vi "rqcBob Channel Test (Low Level Example).vi"() -> ()   [LabVIEW 2019]
uses:
  FPGA/rqcBob/Custom Controls/Pulse Train/rqcBob Pulse Train Config.ctl
  FPGA/rqcBob/Custom Controls/Pulse Train/rqcBob Pulse Train.Generation Mode.ctl
  FPGA/rqcBob/Custom Controls/Pulse Train/rqcBob Pulse Train.First Pulse Delay Mode.ctl
  FPGA/rqcBob/Custom Controls/rqcBob Modulator Config.ctl
  FPGA/rqcBob/Custom Controls/rqcBob Window Config.ctl
  Shared/Shared FPGA Lib/Shared Logic/Custom Controls/rqc Random Generator.parameters.ctl
  Shared/Shared FPGA Lib/Shared Logic/Custom Controls/rqc Random Generator.value type.ctl
  FPGA/rqcBob/Custom Controls/rqcBob Trigger Type.ctl
  <vilib>/FPGAPlugInAG/PCIe-7820R/niLvFpga_Open_PCIe-7820R.vi
  <vilib>/rvi/interface/common/dynamic/niFpgaDynamicAddResources.vi
  Low Level API/Configuration/Photon Detector/Detection FIFOs config/rqcBob Configure PD Detect FIFO (1PD PD1).vi
  Low Level API/Read/Read PD Detection FIFO/rqcBob Read PD Detection FIFO (1PD PD1).vi
  <vilib>/FPGAPlugInAG/Dynamic/niLvFpga_Close_Dynamic.vi
  <vilib>/rvi/interface/nirviOpenFPGA/nirviOpenFPGA.xnode
  FPGA Bitfiles/rqcBob (FPGA) 7820  (MB_SPARTAN7) v 4.0.0.lvbitx.lvbitx
  <vilib>/rvi/interface/nirviCloseFPGA/nirviCloseFPGA.xnode
  <vilib>/Analysis/NI_AALPro.lvlib
panel:
  out "Histogram graph":T1(graph)
  out "Done":bool=TRUE
  in  "stop":bool
  in  "Tab Control":T2(tab)
  in  "train.configuration":T3={"period"=0, "num of pulses"=0, "mode"=enum."train sequence.single", "num of trains"=0, "first pulse delay mode"=enum."every train", "first pulse delay"=55} caption="Pulsed laser configuration"
  in  "modulator.config":T6 caption="Phase modulation"
  in  "window.config":T7 caption="Registration of detector clicks"
  in  "rndGen.parameters":T8={"value type"=enum."constant", "constant"=0, "num of levels"=4, "levels values"=[0, 0, 0, 0]} caption="Phase modulation value" {"num of levels" min=4 max=4 step=1}
  out "Parameters Check Msg":string="Selected parameter combination\nmay lead to inappropriate measurement results"
  in  "Blank Button":bool
  out "sum":i32 caption="Total detector clicks"
  out "DRC":dbl=nan caption="Detection Clicks Rate (Clicks/sec)"
  in  "modulator.clock delay":fxp<+,4,4> caption="PM Clock Delay (0-7) (in units of 40ns)"
  out "SPD.max meas length":u32 caption="SPD max measurement length (in units of 5ns)"
  in  "train.software trigger":bool
  # "Constant"
  # "Random"
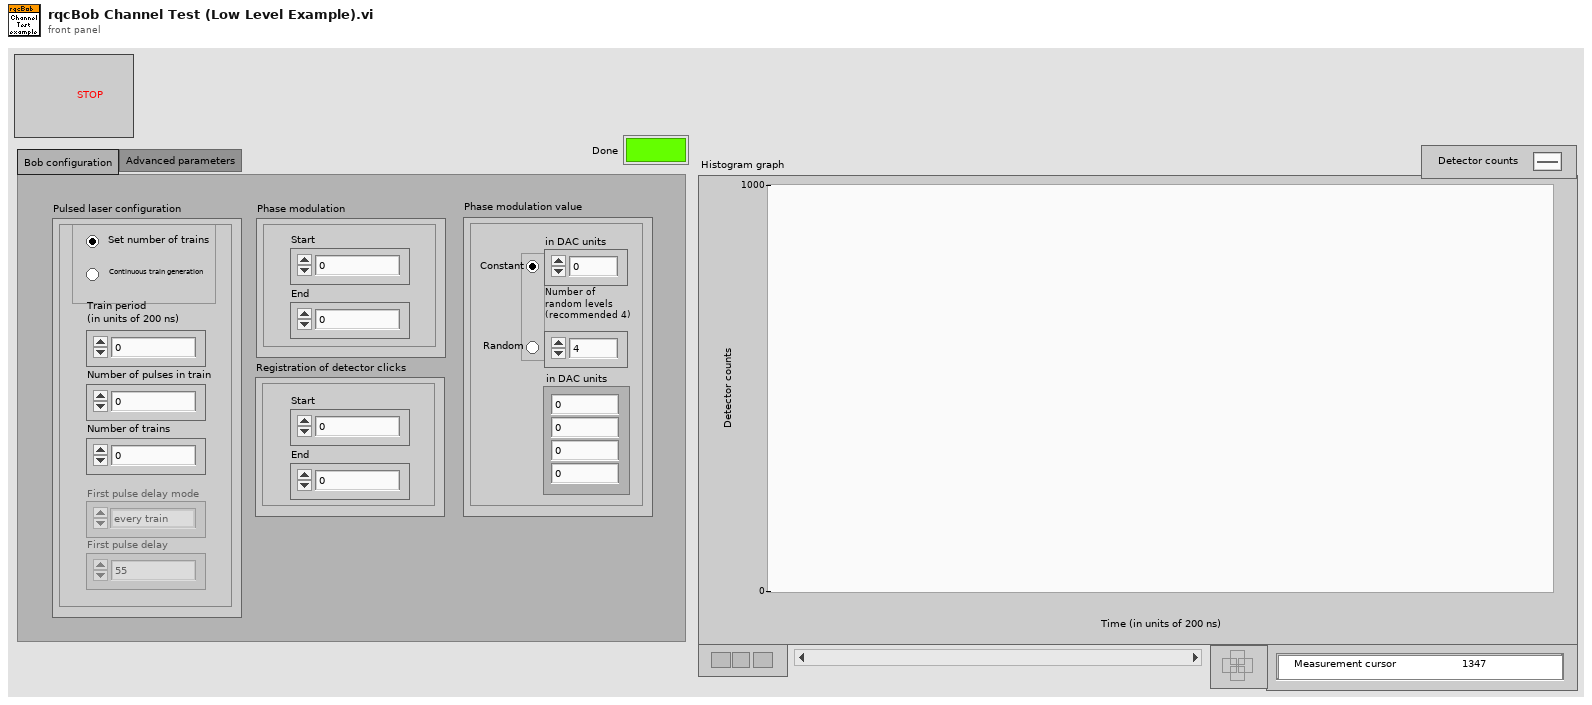
[diagram p1: front panel]
types:
  T1 = cluster{"X Values":dbl[], "Histogram: h(x)":i32[]}
  T2 = enum32{"Bob configuration", "Advanced parameters"}
  T3 = typedef "rqcBob Pulse Train Config.ctl" = cluster{"period":u16, "num of pulses":u16, "mode":T4, "num of trains":u16, "first pulse delay mode":T5, "first pulse delay":u16}
  T4 = typedef "rqcBob Pulse Train.Generation Mode.ctl" = enum32{"single train", "train sequence.single", "train sequence.wait for trigger", "continuous"}
  T5 = typedef "rqcBob Pulse Train.First Pulse Delay Mode.ctl" = enum8{"none", "every train", "first train"}
  T6 = typedef "rqcBob Modulator Config.ctl" = cluster{"modulator.start":u16, "modulator.stop":u16}
  T7 = typedef "rqcBob Window Config.ctl" = cluster{"window.open":u16, "window.close":u16}
  T8 = typedef "rqc Random Generator.parameters.ctl" = cluster{"value type":T9, "constant":u16, "num of levels":u16, "levels values":u16[]}
  T9 = typedef "rqc Random Generator.value type.ctl" = enum32{"random value", "constant"}
  T10 = typedef "rqcBob Trigger Type.ctl" = enum16{"software", "immediate", "DIO"}
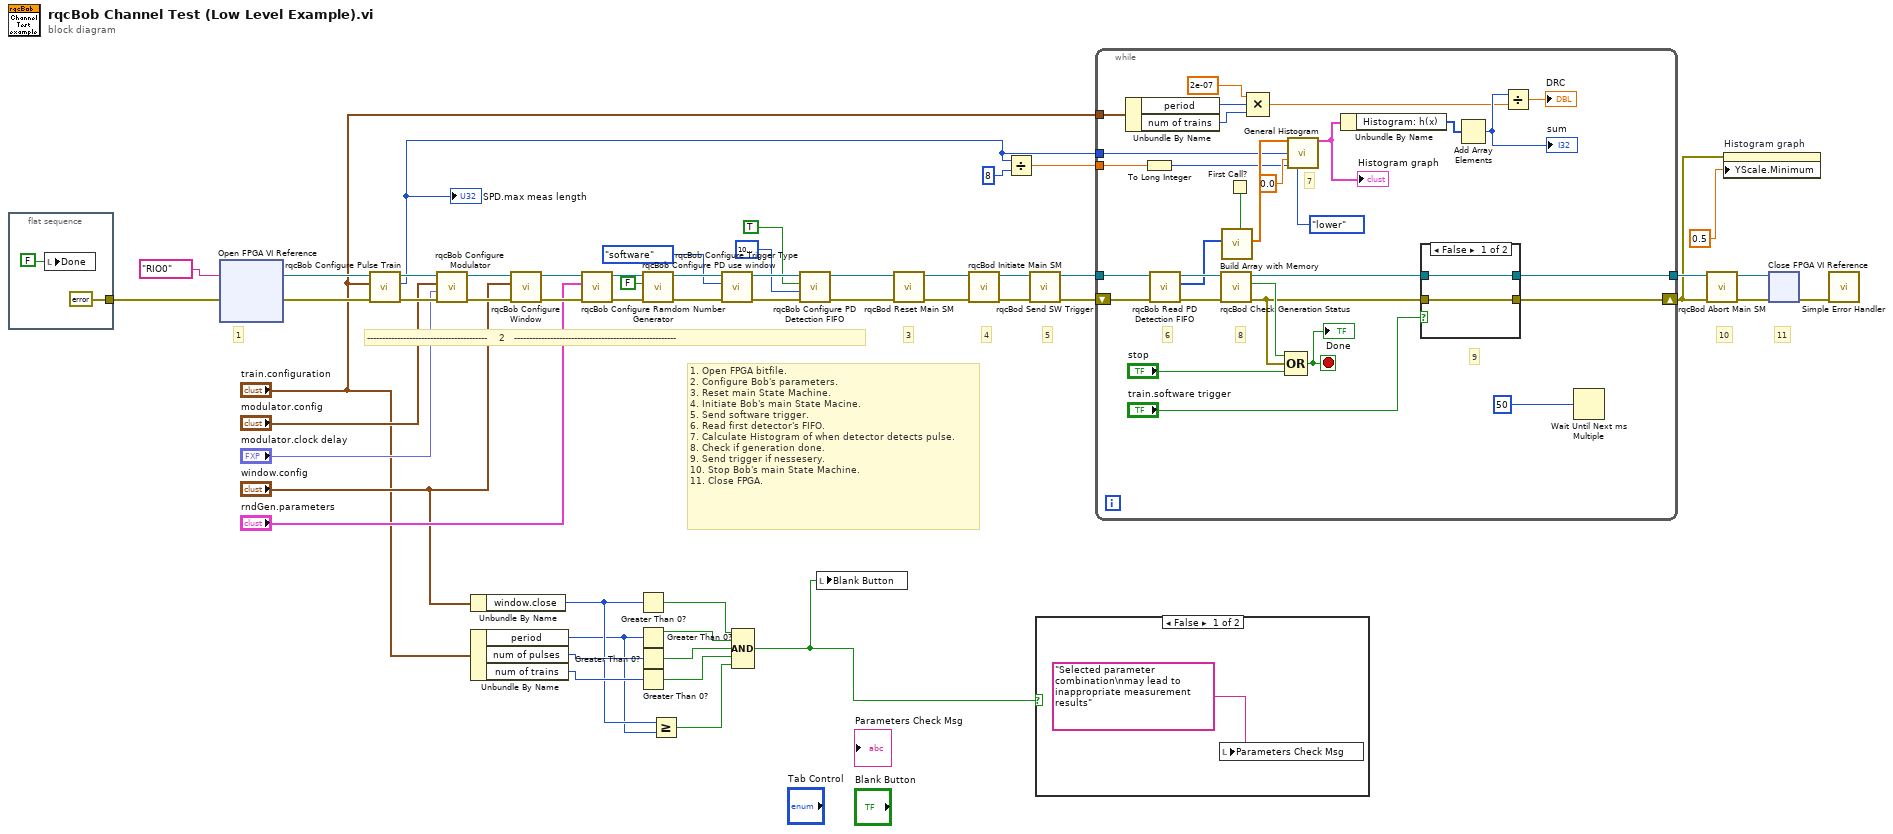
[diagram p0: block diagram]
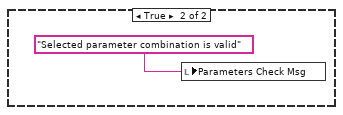
[diagram p2: hidden frame]
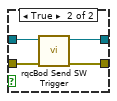
[diagram p3: hidden frame]
diagram:
  # "1. Open FPGA bitfile.\n2. Configure Bob's parameters.\n3. Reset main State Machine.\n4. Initiate Bob's main State Macine.\n5. Send software trigger.\n6. Read first detector's FIFO.\n7. Calculate Histogram of when detector detects pulse.\n8. Check if generation done.\n9. Send trigger if nessesery.\n10. Stop Bob's main State Machine.\n11. Close FPGA."
  # "1"
  # "11"
  # "10"
  # "5"
  # "4"
  # "3"
  # "----------------------------------------    2   ------------------------------------------------------"
  n1 = flat-sequence {
    tunnel: [errorcluster {"status"=FALSE, "code"=0, "source"=""} ("error in")] -> w31
    frame #0 {
      n2 = local write "Done"(FALSE ("Done")) -> ()
    }
  }
  n3 = xnode "Open FPGA VI Reference"("error in"=w31, "resource name"=tag "RIO0") -> ("FPGA VI Reference Out"=w28:refnum<k20>, "error out"=w27:errorcluster)
  n4 = call "rqcBob Configure Pulse Train.vi"("error in"=w27, "train.configuration"="train.configuration", "FPGA reference in"=w28) -> ("error out"=w50:errorcluster, "SPD meas length"=w3:u32, "FPGA reference out"=w51:refnum<k20>)  [unwired: 6 in]
  "SPD.max meas length" <- w3
  n5 = call "rqcBob Configure Modulator.vi"("error in"=w50, "modulator.clock delay"="modulator.clock delay", "modulator.config"="modulator.config", "FPGA reference in"=w51) -> ("error out"=w47:errorcluster, "FPGA reference out"=w48:refnum<k20>)  [unwired: 6 in]
  n6 = Unbundle By Name("window.config") -> ("window.close"=w9:u16)
  n7 = Unbundle By Name("train.configuration") -> ("period"=w8:u16, "num of pulses"=w15:u16, "num of trains"=w14:u16)
  n8 = call "rqcBob Configure Window.vi"("error in"=w47, "window.config"="window.config", "FPGA reference in"=w48) -> ("error out"=w45:errorcluster, "FPGA reference out"=w46:refnum<k20>)  [unwired: 7 in]
  n9 = call "rqcBob Configure Ramdom Number Generator.vi"("error in"=w45, "rqcBob rndGen.parameters"="rndGen.parameters", "FPGA reference in"=w46) -> ("error out"=w44:errorcluster, "FPGA reference out"=w43:refnum<k20>)  [unwired: 7 in]
  n10 = Greater Than 0?(x=w9) -> (x > 0?=w10:bool)
  n11 = Greater Than 0?(x=w8) -> (x > 0?=w11:bool)
  n12 = Greater Than 0?(x=w15) -> (x > 0?=w13:bool)
  n13 = Greater Than 0?(x=w14) -> (x > 0?=w12:bool)
  n14 = call "rqcBob Configure PD use window.vi"("error in"=w44, "PD.use window"=FALSE ("SPD.use detector window"), "FPGA reference in"=w43) -> ("error out"=w41:errorcluster, "FPGA reference out"=w42:refnum<k20>)  [unwired: 7 in]
  n15 = Greater Or Equal?(x=w9, y=w8) -> (x >= y?=w7:bool)
  n16 = call "rqcBob Configure Trigger Type.vi"("error in"=w41, "rqcBob Trigger Type"=rqcBob_Trigger_Type."software", "FPGA reference in"=w42) -> ("error out"=w23:errorcluster, "FPGA reference out"=w25:refnum<k20>)  [unwired: 7 in]
  n17 = Compound Arithmetic op=AND(w10, w11, w13, w12, w7) -> (w6:bool)
  n18 = call-poly "rqcBob Configure PD Detection FIFO.vi"("error in"=w23, "PD.detect fifo depth"=u32 1000000 ("SPD.detect fifo depth"), "PD.detect fifo write enable"=TRUE ("SPD.detect fifo write enable"), "FPGA reference in"=w25) -> ("error out"=w22:errorcluster, "FPGA reference out"=w24:refnum<k20>)  [unwired: 6 in]
  n19 = local write "Blank Button"(w6) -> ()
  n20 = call "rqcBod Reset Main SM.vi"("error in"=w22, "FPGA reference in"=w24) -> ("error out"=w38:errorcluster, "FPGA reference out"=w39:refnum<k20>)  [unwired: 8 in]
  n21 = call "rqcBod Initiate Main SM.vi"("error in"=w38, "FPGA reference in"=w39) -> ("error out"=w36:errorcluster, "FPGA reference out"=w37:refnum<k20>)  [unwired: 8 in]
  n22 = Divide(x=w3, y=u32 8) -> (x/y=w5:dbl)
  n23 = call "rqcBod Send SW Trigger.vi"("error in"=w36, "FPGA reference in"=w37) -> ("error out"=w34:errorcluster, "FPGA reference out"=w35:refnum<k20>)  [unwired: 8 in]
  n24 = case shown="False" w6 {
    frame False {
      n25 = local write "Parameters Check Msg"("Selected parameter combination\nmay lead to inappropriate measurement results") -> ()
    }
    frame True {
      n26 = local write "Parameters Check Msg"("Selected parameter combination is valid") -> ()
    }
  }
  n27 = while {
    tunnel: w35 -> [w77]
    shift-right: [w83] -> w1
    shift-left: w34 -> [w74]
    tunnel: w5 -> [w58]
    tunnel: [w82] -> w19
    tunnel: "train.configuration" -> [w72]
    tunnel: w3 -> [w62]
    stop <- w80 stop-if-true
    # "7"
    # "9"
    # "8"
    # "6"
    n28 = Unbundle By Name(w72) -> ("period"=w71:u16, "num of trains"=w69:u16)
    n29 = To Long Integer(number=w58) -> (32bit integer=w57:i32)
    n30 = call-poly "rqcBob Read PD Detection FIFO.vi"("error in"=w74, "FPGA reference in"=w77) -> ("error out"=w73:errorcluster, "Data"=w75:u32[], "FPGA reference out"=w76:refnum<k20>)  [unwired: 6 in, 1 out]
    n31 = call "rqcBod Check Generation Status.vi"("error in"=w73, "FPGA reference in"=w76) -> ("error out"=w65:errorcluster, "generation.done"=w85:bool, "FPGA reference out"=w84:refnum<k20>)  [unwired: 7 in]
    n32 = First Call?() -> (First Call?: T/F=w78:bool)
    n33 = call "Build Array with Memory.vi"("reset"=w78, "new array"=w75) -> ("appended array"=w64:dbl[])  [unwired: 9 in]
    n34 = Compound Arithmetic op=MULTIPLY(2e-07, w71, w69) -> (w67:dbl)
    n35 = Compound Arithmetic op=OR(w85, w65, "stop") -> (w80:bool)
    "Done" <- w80
    n36 = call <vilib>:"General Histogram.vi"("X"=w64, "max"=w62, "min"=0.0, "# bins"=w57, "inclusion"=enum32{"lower", "upper"}."lower") -> ("Histogram Graph"=w60:T1)  [unwired: 6 in, 4 out]
    "Histogram graph" <- w60
    n37 = Unbundle By Name(w60) -> ("Histogram: h(x)"=w59:i32[])
    n38 = case shown="False" "train.software trigger" {
      tunnel: w84 -> [w88 w92]
      tunnel: w65 -> [w87 w91]
      tunnel: [w88 w90] -> w82
      tunnel: [w87 w89] -> w83
      frame False {
      }
      frame True {
        n39 = call "rqcBod Send SW Trigger.vi"("error in"=w91, "FPGA reference in"=w92) -> ("error out"=w89:errorcluster, "FPGA reference out"=w90:refnum<k20>)  [unwired: 8 in]
      }
    }
    n40 = Add Array Elements(numeric array=w59) -> (sum=w68:i32)
    "sum" <- w68
    n41 = Divide(x=w68, y=w67) -> (x/y=→"DRC":dbl)
    n42 = Wait Until Next ms Multiple(millisecond multiple=u32 50) -> ()  [unwired: 1 out]
  }
  n43 = call "rqcBod Abort Main SM.vi"("error in"=w1, "FPGA reference in"=w19) -> ("error out"=w32:errorcluster, "FPGA reference out"=w33:refnum<k20>)  [unwired: 8 in]
  n44 = property on="Histogram graph" class="XYGraph (strict)"(error in=w1, "YScale.Minimum"=0.5 ("Y Scale.Range:Minimum")) -> ()  [unwired: 1 in, 2 out]
  n45 = xnode "Close FPGA VI Reference"("FPGA VI Reference In"=w33, "error in"=w32) -> ("error out"=w30:errorcluster)
  n46 = call <vilib>:"Simple Error Handler.vi"("error in (no error)"=w30) -> ()  [unwired: 4 in, 5 out]
